vi "Get Waveform Streams for Data Event.vi"   [LabVIEW 2020, in "NI_VS Waveform Streaming Interface.lvlib"]
doc: "Returns references to all waveform stream specifications for which you previously registered for events. Wire data to the <B>registered waveform data event (DBL) in</B> input to determine the polymorphic instance to use or manually select the instance."
uses:
  <vilib>/NI VeriStand/Execution/WaveformStreaming/NI_VS Waveform Streaming Interface.lvlib
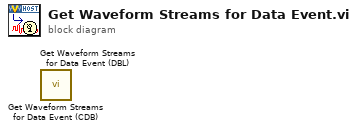
[diagram p0: block diagram]
diagram:
  n1 = call <vilib>:"Get Waveform Streams for Data Event (CDB).vi"() -> ()  [unwired: 9 in, 3 out]
  n2 = call <vilib>:"Get Waveform Streams for Data Event (DBL).vi"() -> ()  [unwired: 9 in, 3 out]
